vi "Destroy Theme.vi"(8 "error in (no error)":errorcluster, 11 "Theme in":refnum<class "Theme.lvclass">) -> (0 "error out":errorcluster)   [LabVIEW 2017, in "Theme.lvlib" / "Theme.lvclass"]
uses:
  Theme.lvclass
  Theme.lvclass/Theme.ctl
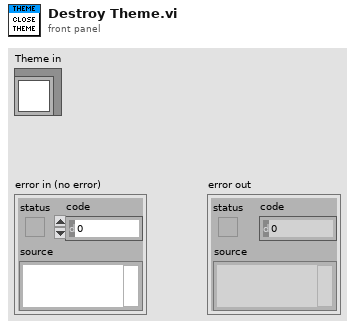
[diagram p1: front panel]
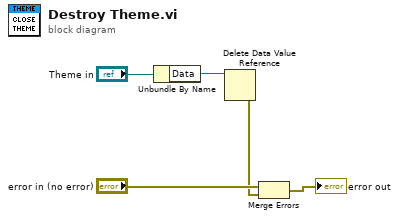
[diagram p0: block diagram]
diagram:
  n1 = Unbundle By Name("Theme in") -> ("Data"=w4:refnum<data-value>)
  n2 = Delete Data Value Reference(data value reference=w4) -> (error out=w1:errorcluster)  [unwired: 1 in, 1 out]
  n3 = Merge Errors("error in (no error)", w1) -> (→"error out":errorcluster)
